vi "Build Package cmd.vi"(0 "Source Path":path, 5 "Destination Dir":path, 11 "error in (no error)":errorcluster) -> (4 "Error Message":string, 15 "error out":errorcluster)   [LabVIEW 2021, in "Measurement Builder.lvlib"]
uses:
  Measurement Builder.lvlib
  Path Functions/Path Functions.lvlib
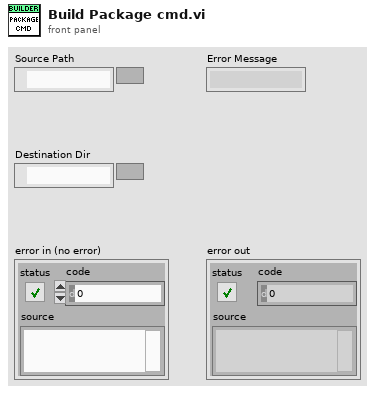
[diagram p1: front panel]
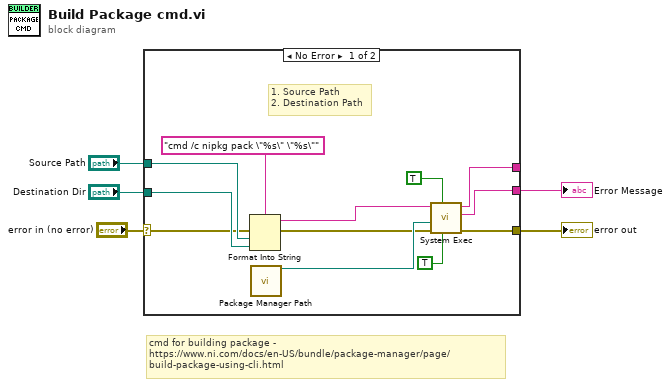
[diagram p0: block diagram]
diagram:
  # "cmd for building package -\nhttps://www.ni.com/docs/en-US/bundle/package-manager/page/build-package-using-cli.html"
  n1 = case shown="No Error" "error in (no error)" {
    selector: "error in (no error)" -> [w8 w18]
    tunnel: [w17 w18] -> w5
    tunnel: "Destination Dir" -> [w16 _]
    tunnel: "Source Path" -> [w15 _]
    tunnel: [w7 _] -> w1
    tunnel: [w6 _] -> _
    frame No Error {
      # "1. Source Path\n2. Destination Path"
      n2 = Format Into String(format string="cmd /c nipkg pack \"%s\" \"%s\"", error in=w8, w15, w16) -> (resulting string=w14:string, error out=w9:errorcluster)  [unwired: 1 in]
      n3 = call "Package Manager Path.vi"() -> ("Package Manager"=w10:path)  [unwired: 15 in]
      n4 = call <vilib>:"System Exec.vi"("run minimized? (F)"=TRUE, "wait until completion? (T)"=TRUE, "error in (no error)"=w9, "working directory"=w10, "command line"=w14) -> ("error out"=w17:errorcluster, "standard error"=w7:string, "standard output"=w6:string)  [unwired: 3 in, 1 out]
    }
    frame Error {
    }
  }
  "error out" <- w5
  "Error Message" <- w1
